vi "ActionVIOnDownload.vi"(5 "System Definition Dir":path, 6 "IP address":string, 7 "Details Ref":refnum<vi>, 8 "error in (no error)":errorcluster, 10 "WebDAV session in":T1, 11 "Device Item Ref in":T2 format="%.0x") -> (0 "error out":errorcluster, 2 "WebDAV session out":T1, 3 "Device Item Ref out":T2 format="%.0x")   [LabVIEW 2018, in "Vires VTD System Explorer.lvlib"]
uses:
  Vires VTD System Explorer.lvlib
  <vilib>/NI Veristand/Custom Device API/Custom Device Item Ref.ctl
  <vilib>/WebDAVClient/Advanced/SessionHandle.ctl
  <vilib>/NI Veristand/Custom Device API/Custom Device API.lvlib
  <vilib>/WebDAVClient/NI_WebDAV.lvlib
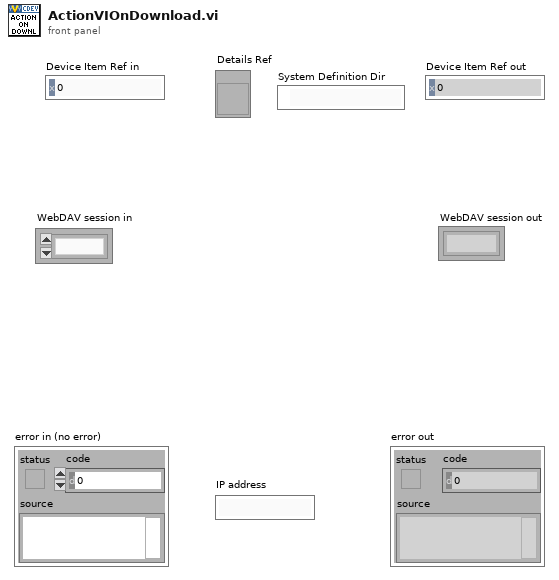
[diagram p1: front panel]
types:
  T1 = typedef "NI_WebDAV.lvlib/SessionHandle.ctl" = refnum<k1>
  T2 = typedef "Custom Device API.lvlib/Custom Device Item Ref.ctl" = u64
  T3 = typedef "Custom Device API.lvlib/Custom Device Target Type.ctl" = enum16{"PharLap", "VxWorks", "Windows", "Linux_32_ARM", "Linux_x64"}
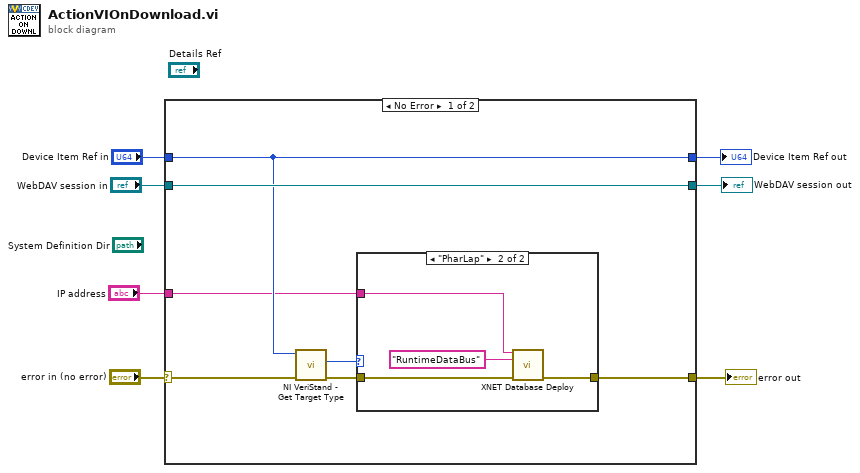
[diagram p0: block diagram]
diagram:
  n1 = case shown="No Error" "error in (no error)" {
    selector: "error in (no error)" -> [w11 w22]
    tunnel: [w9 w22] -> w6
    tunnel: "WebDAV session in" -> [w14 w21]
    tunnel: [w14 w21] -> w2
    tunnel: "Device Item Ref in" -> [w10 w20]
    tunnel: [w10 w20] -> w4
    tunnel: "IP address" -> [w8 _]
    frame No Error {
      n2 = call <vilib>:"NI VeriStand - Get Target Type.vi"("error in (no error)"=w11, "Item Ref in"=w10) -> ("error out"=w12:errorcluster, "Target Type"=w13:T3)  [unwired: 7 in, 1 out]
      n3 = case shown="\"PharLap\"" w13 {
        tunnel: w8 -> [_ w18]
        tunnel: w12 -> [w15 w17]
        tunnel: [w15 w16] -> w9
        frame Default {
        }
        frame "PharLap" {
          n4 = call <vilib>:"XNET Database Deploy.vi"("IP address"=w18, "alias"="RuntimeDataBus", "error in (no error)"=w17) -> ("error out"=w16:errorcluster)  [unwired: 11 in, 1 out]
        }
      }
    }
    frame Error {
    }
  }
  "error out" <- w6
  "Device Item Ref out" <- w4
  "WebDAV session out" <- w2
